vi "CaptStubSaturation.vi"(6 "Graph in":cluster{dbl[], dbl[]}, 7 "Index":i32, 8 "error in":errorcluster, 9 "Length":i32=250, 11 "ON":bool) -> (0 "error out":errorcluster, 2 "Values":cluster{dbl[], dbl[]})   [LabVIEW 2012]
uses:
  GlobalVariables/CalibrationState.vi
  GlobalVariables/CalibrationVolumes.vi
  GlobalVariables/Samples.vi
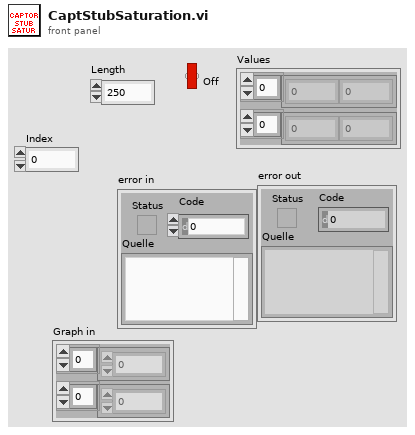
[diagram p1: front panel]
types:
  T1 = cluster{"Pressure":cluster{"TimeSamples":dbl[], "PressureSamples":dbl[]}, "Flow":cluster{"TimeSamples":dbl[], "FlowSamples":dbl[]}}
  T2 = cluster{"CalibrationVolumes":dbl[], "SetName":string}[]
  T3 = cluster{bool, "CalibrationStep":u32, "PressureCons":dbl[], "PressureMes":dbl[], "Weights":bool[], "CalibrationCaptor":u32}
  T4 = cluster{"TimeSamples":dbl[], "PressureSamples":dbl[]}
  T5 = cluster{"TimeSamples":dbl[], "FlowSamples":dbl[]}
  T6 = cluster{cluster{"TimeSamples":dbl[], "PressureSamples":dbl[]}, "Flow":cluster{"TimeSamples":dbl[], "FlowSamples":dbl[]}}
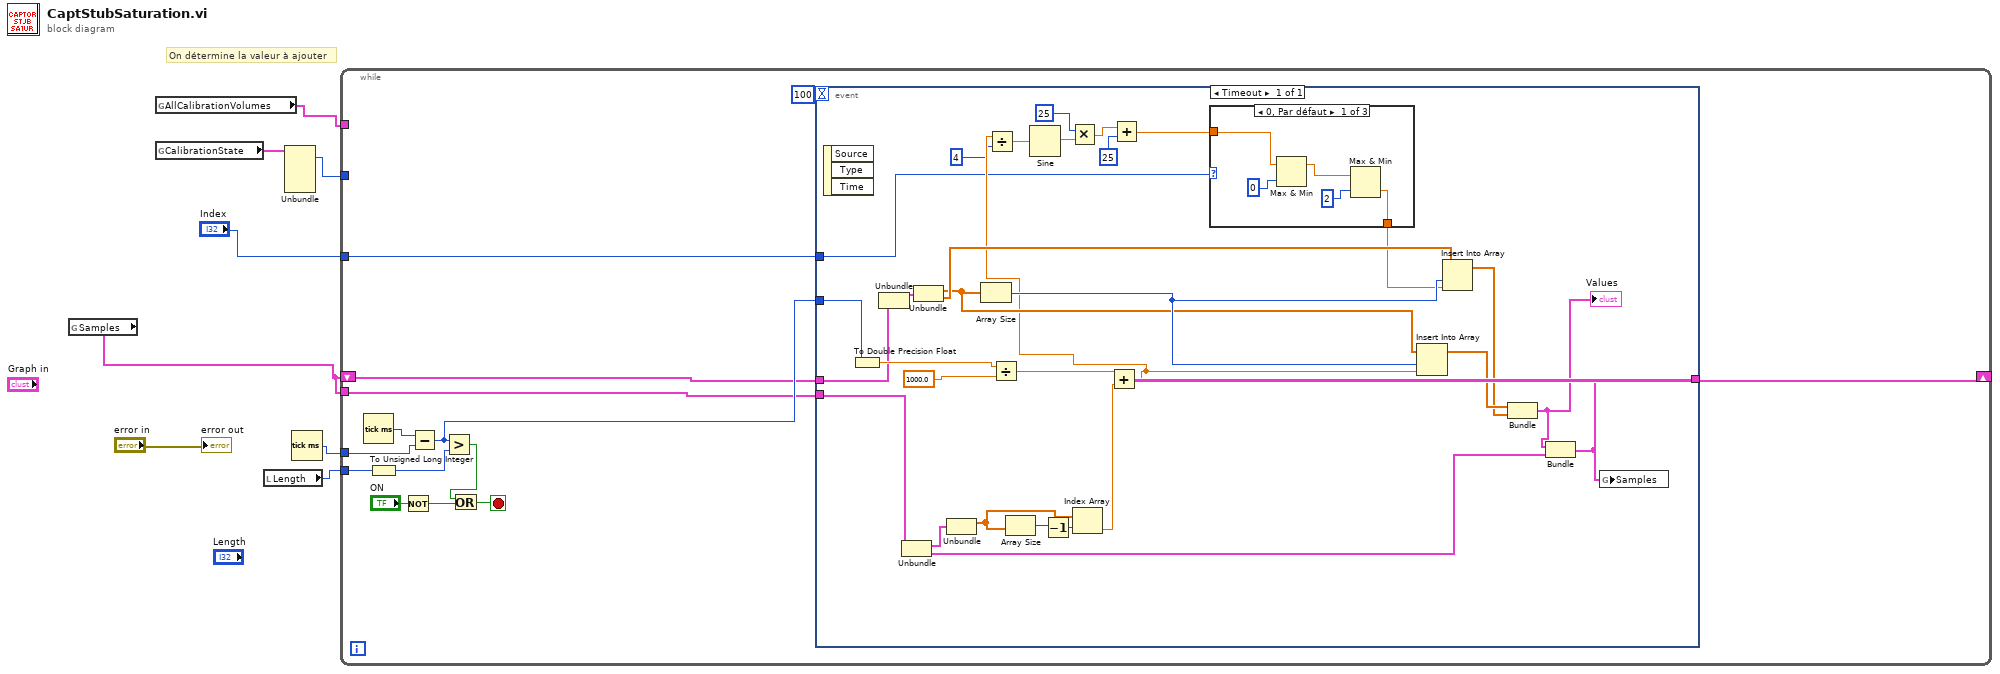
[diagram p0: block diagram]
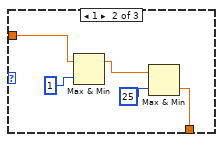
[diagram p2: hidden frame]
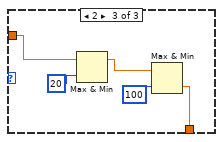
[diagram p3: hidden frame]
diagram:
  # "On détermine la valeur à ajouter"
  n1 = global read "Samples.vi" "Samples"() -> (w2:T1)
  n2 = global read "CalibrationVolumes.vi" "AllCalibrationVolumes"() -> (w4:T2)
  n3 = global read "CalibrationState.vi" "CalibrationState"() -> (w5:T3)
  n4 = local read "Length"() -> (w7:i32)
  n5 = Unbundle(w5) -> ("CalibrationStep"=w3:u32)  [unwired: 5 out]
  n6 = Tick Count (ms)() -> (millisecond timer value=w8:u32)
  n7 = while {
    tunnel: w8 -> [w18]
    tunnel: w7 -> [w13]
    shift-right: [w11] -> _
    shift-left: w2 -> [w14]
    tunnel: w4 -> [_]
    tunnel: w3 -> [_]
    tunnel: w2 -> [w10]
    tunnel: "Index" -> [w9]
    stop <- w20 stop-if-true
    n8 = Tick Count (ms)() -> (millisecond timer value=w19:u32)
    n9 = To Unsigned Long Integer(number=w13) -> (unsigned 32bit integer=w12:u32)
    n10 = Not(x="ON") -> (.not. x?=w21:bool)
    n11 = Subtract(x=w19, y=w18) -> (x-y=w15:u32)
    n12 = Greater?(x=w15, y=w12) -> (0:w17:bool)
    n13 = Or(x=w17, y=w21) -> (x .or. y?=w20:bool)
    n14 = event shown="[0] Timeout" {
      selector: _ -> [_]
      dyn-events: _ -> [_]
      timeout: 100 -> [_]
      tunnel: w15 -> [w48]
      tunnel: w14 -> [w45]
      tunnel: [w33] -> w11
      tunnel: w10 -> [w44]
      tunnel: w9 -> [w25]
      event Timeout {
        n15 = event-data() -> ()  [unwired: 1 in, 3 out]
        n16 = To Double Precision Float(number=w48) -> (double precision float=w47:dbl)
        n17 = Unbundle(w45) -> ("Pressure"=w37:T4)  [unwired: 1 out]
        n18 = Unbundle(w44) -> ("Pressure"=w39:T4, "Flow"=w34:T5)
        n19 = Unbundle(w37) -> ("TimeSamples"=w36:dbl[], "PressureSamples"=w38:dbl[])
        n20 = Unbundle(w39) -> ("TimeSamples"=w40:dbl[])  [unwired: 1 out]
        n21 = Array Size(array=w36) -> (size(s)=w43:i32)
        n22 = Divide(x=w47, y=1000.0) -> (x/y=w49:dbl)
        n23 = Array Size(array=w40) -> (size(s)=w52:i32)
        n24 = Decrement(x=w52) -> (x-1=w51:i32)
        n25 = Index Array(array=w40, index=w51) -> (element=w46:dbl)
        n26 = Add(x=w49, y=w46) -> (x+y=w28:dbl)
        n27 = Divide(x=w28, y=4) -> (x/y=w27:dbl)
        n28 = Sine(x=w27) -> (sin(x)=w31:dbl)
        n29 = Multiply(x=25, y=w31) -> (x*y=w30:dbl)
        n30 = Add(x=w30, y=25) -> (x+y=w24:dbl)
        n31 = case shown="0, Par défaut" w25 {
          tunnel: w24 -> [w57 w59 w64]
          tunnel: [w53 w58 w63] -> w23
          frame 0, Default {
            n32 = Max & Min(x=w57, y=0) -> (max(x,y)=w54:dbl)  [unwired: 1 out]
            n33 = Max & Min(x=w54, y=2) -> (min(x,y)=w53:dbl)  [unwired: 1 out]
          }
          frame 1 {
            n34 = Max & Min(x=w59, y=1) -> (max(x,y)=w60:dbl)  [unwired: 1 out]
            n35 = Max & Min(x=w60, y=25) -> (min(x,y)=w58:dbl)  [unwired: 1 out]
          }
          frame 2 {
            n36 = Max & Min(x=w64, y=20) -> (max(x,y)=w65:dbl)  [unwired: 1 out]
            n37 = Max & Min(x=w65, y=100) -> (min(x,y)=w63:dbl)  [unwired: 1 out]
          }
        }
        n38 = Insert Into Array(array=w36, index=w43, new element=w28) -> (w42:dbl[])
        n39 = Insert Into Array(array=w38, index=w43, new element=w23) -> (w41:dbl[])
        n40 = Bundle("TimeSamples"=w42, "PressureSamples"=w41) -> (w35:T4)  [unwired: 1 in]
        "Values" <- w35
        n41 = Bundle(w35, "Flow"=w34) -> (w33:T6)  [unwired: 1 in]
        n42 = global write "Samples.vi" "Samples"(w33) -> ()
      }
    }
  }
  "error out" <- "error in"
